vi "SP Remove Adapter Effects.vi"(8 "error in (no error)":errorcluster, 9 "Adapter S Parameters":T1, 10 "Data S Parameters":T1, 11 "Multiplication Order":enum16{"Adapter * Data", "Data * Adapter"}(ring)) -> (0 "error out":errorcluster, 2 "New Data  S Parameters":T1)   [LabVIEW 2011]
uses:
  TypeDefs/SP Data.ctl
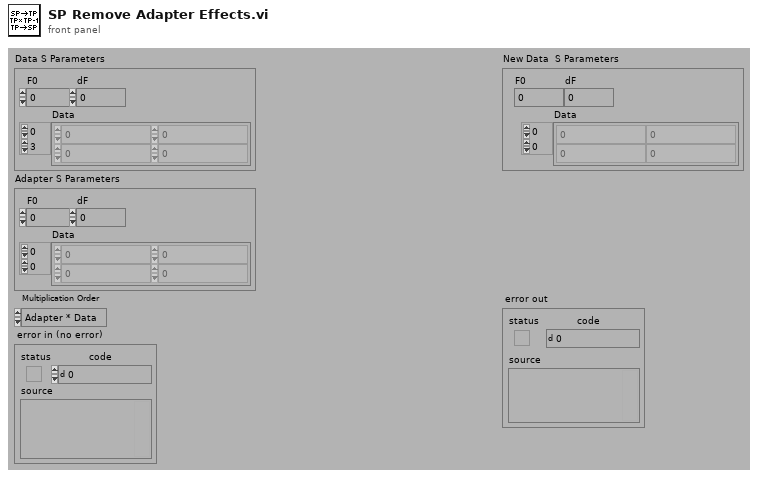
[diagram p1: front panel]
types:
  T1 = typedef "SP Data.ctl" = cluster{"F0":dbl, "dF":dbl, "Data":cdb[][]}
  T2 = typedef "SP TP Data.ctl" = cluster{"F0":dbl, "dF":dbl, "Data":cdb[][][]}
  T3 = typedef "SP Complex Matrix.ctl" = cdb[][]
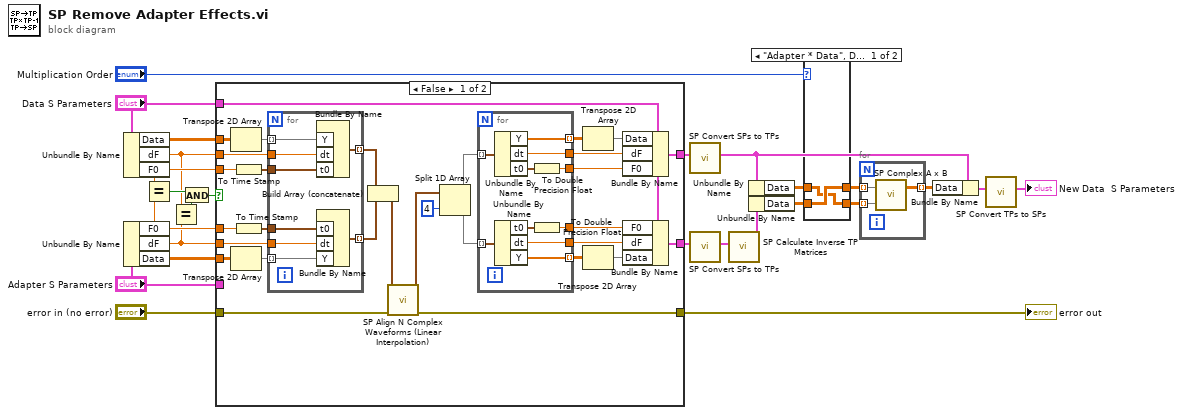
[diagram p0: block diagram]
diagram:
  n1 = Unbundle By Name("Data S Parameters") -> ("Data"=w23:cdb[][], "dF"=w18:dbl, "F0"=w19:dbl)
  n2 = Unbundle By Name("Adapter S Parameters") -> ("F0"=w21:dbl, "dF"=w20:dbl, "Data"=w22:cdb[][])
  n3 = Equal?(x=w19, y=w21) -> (x = y?=w25:bool)
  n4 = Equal?(x=w18, y=w20) -> (x = y?=w26:bool)
  n5 = And(x=w25, y=w26) -> (x .and. y?=w24:bool)
  n6 = case shown="False" w24 {
    tunnel: w23 -> [w55 _]
    tunnel: w22 -> [w38 _]
    tunnel: w21 -> [w30 _]
    tunnel: w20 -> [w54 _]
    tunnel: w19 -> [w28 _]
    tunnel: w18 -> [w56 _]
    tunnel: "error in (no error)" -> [w32 w77]
    tunnel: [w31 w77] -> w16
    tunnel: "Data S Parameters" -> [w42 w75]
    tunnel: [w41 w75] -> w13
    tunnel: [w40 w76] -> w12
    tunnel: "Adapter S Parameters" -> [_ w76]
    frame False {
      n7 = Transpose 2D Array(2D array=w55) -> (transposed array=w39:cdb[][])
      n8 = Transpose 2D Array(2D array=w38) -> (transposed array=w37:cdb[][])
      n9 = To Time Stamp(1:w28) -> (0:w27:timestamp)
      n10 = To Time Stamp(1:w30) -> (0:w29:timestamp)
      n11 = for {
        tunnel: w56 -> [w74]
        tunnel: w39 -> [w73] mode=indexing
        tunnel: w54 -> [w72]
        tunnel: w37 -> [w71] mode=indexing
        tunnel: [w70] -> w52 mode=indexing
        tunnel: [w69] -> w53 mode=indexing
        tunnel: w29 -> [w68]
        tunnel: w27 -> [w67]
        n12 = Bundle By Name("Y"=w73, "dt"=w74, "t0"=w67) -> (w70:waveform(cdb))  [unwired: 1 out]
        n13 = Bundle By Name("t0"=w68, "dt"=w72, "Y"=w71) -> (w69:waveform(cdb))  [unwired: 1 out]
      }
      n14 = Build Array (concatenate)(w52, w53) -> (w51:waveform(cdb)[])
      n15 = call "SP Align N Complex Waveforms (Linear Interpolation).vi"("error in (no error)"=w32, "Waveforms In"=w51) -> ("error out"=w31:errorcluster, "Aligned Waveforms In"=w50:waveform(cdb)[])  [unwired: 3 in, 5 out]
      n16 = Split 1D Array(array=w50, index=4) -> (first subarray=w48:waveform(cdb)[], second subarray=w47:waveform(cdb)[])
      n17 = for {
        tunnel: w48 -> [w66] mode=indexing
        tunnel: w47 -> [w65] mode=indexing
        tunnel: [w62] -> w46
        tunnel: [w61] -> w43
        tunnel: [w60] -> w45
        tunnel: [w59] -> w44
        tunnel: [w58] -> w33 mode=indexing
        tunnel: [w57] -> w36 mode=indexing
        n18 = Unbundle By Name(w66) -> ("Y"=w58:cdb[], "dt"=w60:dbl, "t0"=w63:timestamp)
        n19 = Unbundle By Name(w65) -> ("t0"=w64:timestamp, "dt"=w59:dbl, "Y"=w57:cdb[])
        n20 = To Double Precision Float(number=w63) -> (double precision float=w62:dbl)
        n21 = To Double Precision Float(number=w64) -> (double precision float=w61:dbl)
      }
      n22 = Transpose 2D Array(2D array=w33) -> (transposed array=w34:cdb[][])
      n23 = Transpose 2D Array(2D array=w36) -> (transposed array=w35:cdb[][])
      n24 = Bundle By Name(cluster=w42, "Data"=w34, "dF"=w45, "F0"=w46) -> (w41:T1)
      n25 = Bundle By Name(cluster=w42, "F0"=w43, "dF"=w44, "Data"=w35) -> (w40:T1)
    }
    frame True {
    }
  }
  "error out" <- w16
  n26 = call "SP Convert SPs to TPs.vi"("SP Array"=w13) -> ("T-Parameters"=w4:T2)  [unwired: 10 out]
  n27 = call "SP Convert SPs to TPs.vi"("SP Array"=w12) -> ("T-Parameters"=w14:T2)  [unwired: 10 out]
  n28 = call "SP Calculate Inverse TP Matrices.vi"("T-Parameters"=w14) -> ("T-Parameters"=w10:T2)  [unwired: 10 out]
  n29 = Unbundle By Name(w4) -> ("Data"=w7:cdb[][][])
  n30 = Unbundle By Name(w10) -> ("Data"=w8:cdb[][][])
  n31 = case shown="\"Adapter * Data\", Default" "Multiplication Order" {
    tunnel: w8 -> [w79 w80]
    tunnel: w7 -> [w78 w81]
    tunnel: [w79 w81] -> w6
    tunnel: [w78 w80] -> w5
    frame "Adapter * Data", Default {
    }
    frame "Data * Adapter" {
    }
  }
  n32 = for {
    tunnel: [w84] -> w3 mode=indexing
    tunnel: w5 -> [w83] mode=indexing
    tunnel: w6 -> [w82] mode=indexing
    n33 = call "SP Complex A x B.vi"("B"=w83, "A"=w82) -> ("A x B"=w84:T3)  [unwired: 1 out]
  }
  n34 = Bundle By Name(cluster=w4, "Data"=w3) -> (w2:T2)
  n35 = call "SP Convert TPs to SPs.vi"("T-Parameters"=w2) -> ("SP Array"=→"New Data  S Parameters":T1)  [unwired: 10 out]
